vi "Read Value.vi"(8 "error in (no error)":errorcluster, 11 "bt_Blackboard Boolean Set in":refnum<class "bt_Blackboard Boolean Set.lvclass">) -> (0 "error out":errorcluster, 2 "Value":bool, 3 "bt_Blackboard Boolean Set out":refnum<class "bt_Blackboard Boolean Set.lvclass">)   [LabVIEW 2021, in "BT.lvlib" / "bt_Blackboard Boolean Set.lvclass"]
uses:
  bt_Blackboard Boolean Set.lvclass
  bt_Blackboard Boolean Set.lvclass/bt_Blackboard Boolean Set.ctl
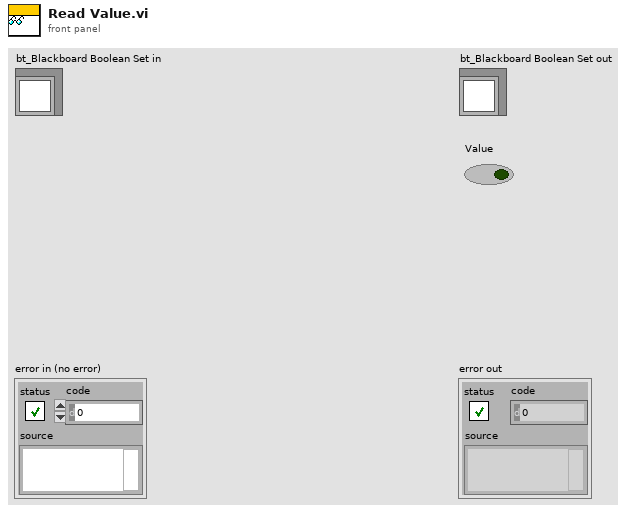
[diagram p1: front panel]
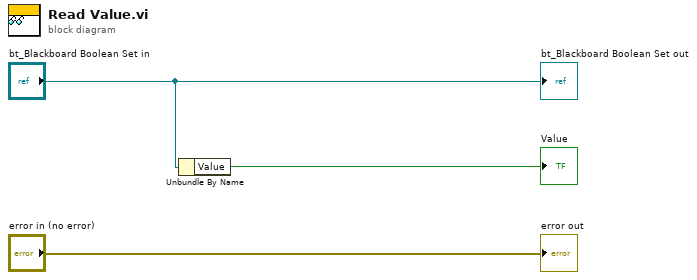
[diagram p0: block diagram]
diagram:
  n1 = Unbundle By Name("bt_Blackboard Boolean Set in") -> ("Value"=→"Value":bool)
  "error out" <- "error in (no error)"
  "bt_Blackboard Boolean Set out" <- "bt_Blackboard Boolean Set in"
